vi "Write_Temp_Data_Log.vi"(6 "Process_time":string, 8 "error in (no error)":errorcluster, 9 "Current (A)":sgl[](array[numeric]), 10 "Voltage (V)":sgl[](array[numeric]), 11 "datalog path (use dialog)":path) -> (0 "error out":errorcluster)   [LabVIEW 2012]
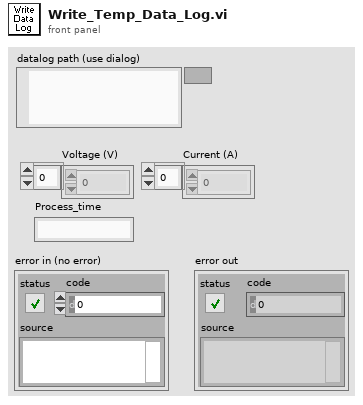
[diagram p1: front panel]
types:
  T1 = enum16{"open", "replace", "create", "open or create", "replace or create", "replace or create with confirmation"}
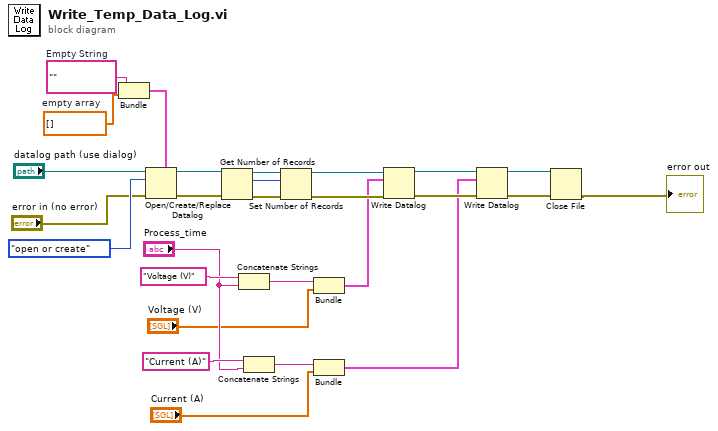
[diagram p0: block diagram]
diagram:
  w27 = ""  # Empty String
  w26 = sgl[] []  # empty array
  n1 = Bundle(w27, "empty array"=w26) -> (w23:cluster{string, "empty array":sgl[]})  [unwired: 1 out]
  n2 = Open/Create/Replace Datalog(5:w23, 8:"error in (no error)", 10:T1."open or create" ("operation (0:open)"), 11:"datalog path (use dialog)") -> (0:w19:errorcluster, 3:w20:refnum<k1>)  [unwired: 3 out]
  n3 = Get Number of Records(4:w19, 7:w20) -> (0:w18:errorcluster, 2:w17:i64, 3:w16:refnum<k1>)
  n4 = Concatenate Strings("Voltage (V)", "Process_time") -> (w7:string)
  n5 = Concatenate Strings("Current (A)", "Process_time") -> (w5:string)
  n6 = Set Number of Records(4:w18, 6:w17, 7:w16) -> (0:w13:errorcluster, 3:w15:refnum<k1>)
  n7 = Bundle(w7, "Voltage (V)"="Voltage (V)") -> (w11:cluster{string, "Voltage (V)":sgl[]})  [unwired: 1 in]
  n8 = Bundle(w5, "Current (A)"="Current (A)") -> (w10:cluster{string, "Current (A)":sgl[]})  [unwired: 1 in]
  n9 = Write Datalog(4:w13, 6:w11, 7:w15) -> (0:w12:errorcluster, 3:w14:refnum<k1>)
  n10 = Write Datalog(4:w12, 6:w10, 7:w14) -> (0:w25:errorcluster, 3:w24:refnum<k1>)
  n11 = Close File(refnum=w24, error in=w25) -> (error out=→"error out":errorcluster)  [unwired: 1 out]
